vi "AWContainerRead.vi"() -> (0 "Output":i16[](array[numeric]))   [LabVIEW 2010, in "Recorder.lvlib"]
uses:
  Recorder.lvlib
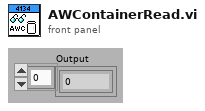
[diagram p1: front panel]
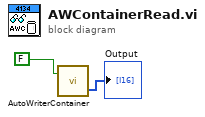
[diagram p0: block diagram]
diagram:
  n1 = call "AutoWriterContainer.vi"("Mode(Write=True)"=FALSE) -> ("Output"=→"Output":i16[])  [unwired: 1 in]
